vi "Lab Panel V5.26.vi"() -> ()   [LabVIEW 2017] (continued)
                n197 = call "sub vi - GET ALL TEMP v7.vi"("LA01-EN"=w245, "simulate"=w207, "LA02-EN"=w245, "LA03-EN"=w245, "LA04-EN"=w245, "LA05-EN"=w245, "Gen Cal Value"=1) -> ("ID"=w206:T24, "LA01 TEMP"=w243:T25, "LA02 TEMP"=w236:T25, "LA03 TEMP"=w229:T25, "LA04 TEMP"=w222:T25, "LA05 TEMP"=w215:T25)  [unwired: 1 in, 2 out]
                n198 = local write "LAB05 TEMP"(w215) -> ()
                n199 = local write "LAB04 TEMP"(w222) -> ()
                n200 = Unbundle(w229) -> ("T1"=w226:dbl, "T2"=w225:dbl, "T3"=w224:dbl, "T4"=w223:dbl)  [unwired: 2 out]
                n201 = Unbundle(w243) -> ("T1"=w241:dbl, "T2"=w240:dbl, "T3"=w239:dbl, "T4"=w238:dbl)  [unwired: 2 out]
                n202 = Unbundle(w236) -> ("T1"=w233:dbl, "T2"=w232:dbl, "T3"=w231:dbl, "T4"=w230:dbl)  [unwired: 2 out]
                n203 = Unbundle(w222) -> ("T1"=w220:dbl, "T2"=w219:dbl, "T3"=w218:dbl, "T4"=w217:dbl)  [unwired: 2 out]
                n204 = Unbundle(w215) -> ("T1"=w213:dbl, "T2"=w212:dbl, "T3"=w211:dbl, "T4"=w210:dbl)  [unwired: 2 out]
                n205 = local write "LAB01 TEMP"(w243) -> ()
                n206 = local write "LAB02 TEMP"(w236) -> ()
                n207 = local write "LAB03 TEMP"(w229) -> ()
                n208 = Unbundle(w206) -> ("id1"=→"LAB01-TP":bool, "id2"=→"LAB02-TP":bool, "id3"=→"LAB03-TP":bool, "id4"=→"LAB04-TP":bool, "id5"=→"LAB05-TP":bool)
                n209 = local read "TEMP LA05"() -> (w214:T9)
                n210 = local read "TEMP LA04"() -> (w221:T9)
                n211 = local read "TEMP LA02"() -> (w235:T9)
                n212 = local read "TEMP LA03"() -> (w228:T9)
                n213 = local read "TEMP LA01"() -> (w242:T9)
                n214 = Bundle(cluster=w228, "TL-1"=w226, "TN-1"=w225, "TL-2"=w224, "TN-2"=w223) -> (w227:T9)  [unwired: 4 in]
                n215 = Bundle(cluster=w242, "TL-1"=w241, "TN-1"=w240, "TL-2"=w239, "TN-2"=w238) -> (w237:T9)  [unwired: 4 in]
                n216 = Bundle(cluster=w235, "TL-1"=w233, "TN-1"=w232, "TL-2"=w231, "TN-2"=w230) -> (w234:T9)  [unwired: 4 in]
                n217 = Bundle(cluster=w221, "TL-1"=w220, "TN-1"=w219, "TL-2"=w218, "TN-2"=w217) -> (w216:T9)  [unwired: 4 in]
                n218 = Bundle(cluster=w214, "TL-1"=w213, "TN-1"=w212, "TL-2"=w211, "TN-2"=w210) -> (w209:T9)  [unwired: 4 in]
                n219 = local write "TEMP LA03"(w227) -> ()
                n220 = local write "TEMP LA01"(w237) -> ()
                n221 = local write "TEMP LA02"(w234) -> ()
                n222 = local write "TEMP LA05"(w209) -> ()
                n223 = local write "TEMP LA04"(w216) -> ()
              }
            }
            frame #2 {
              w256 = 0
              n224 = local read "LAB01 TEMP"() -> (w258:T12)
              n225 = local read "SIG LAB01-2"() -> (w253:T2)
              n226 = Unbundle By Name(w258) -> ("T1 Live"=w251:dbl, "T1 Neut"=w250:dbl, "T2 Live"=w249:dbl, "T2 Neut"=w248:dbl)  [unwired: 2 out]
              n227 = local read "SIG LAB01-1"() -> (w255:T2)
              n228 = local read "TEMP LA01"() -> (w259:T9)
              n229 = Bundle By Name(cluster=w259, "TL-1"=w251, "TN-1"=w250, "TL-2"=w249, "TN-2"=w248, "TL -1COUNT"=w256, "TN-1 COUNT"=w256, "TL-2 COUNT"=w256, "TN-2 COUNT"=w256) -> (w257:T9)
              n230 = Bundle(cluster=w255, "Tmp Live"=w251, "Tmp Neut"=w250) -> (w254:T2)  [unwired: 3 in]
              n231 = Bundle(cluster=w253, "Tmp Live"=w249, "Tmp Neut"=w248) -> (w252:T2)  [unwired: 3 in]
              n232 = local write "SIG LAB01-2"(w252) -> ()
              n233 = local write "SIG LAB01-1"(w254) -> ()
              n234 = local write "TEMP LA01"(w257) -> ()
            }
            frame #3 {
              w268 = 0
              n235 = local read "LAB02 TEMP"() -> (w270:T12)
              n236 = Unbundle By Name(w270) -> ("T1 Live"=w263:dbl, "T1 Neut"=w262:dbl, "T2 Live"=w261:dbl, "T2 Neut"=w260:dbl)  [unwired: 2 out]
              n237 = local read "SIG LAB02-1"() -> (w267:T2)
              n238 = local read "SIG LAB02-2"() -> (w266:T2)
              n239 = local read "TEMP LA02"() -> (w271:T9)
              n240 = Bundle By Name(cluster=w271, "TL-1"=w263, "TN-1"=w262, "TL-2"=w261, "TN-2"=w260, "TL -1COUNT"=w268, "TN-1 COUNT"=w268, "TL-2 COUNT"=w268, "TN-2 COUNT"=w268) -> (w269:T9)
              n241 = Bundle(cluster=w266, "Tmp Live"=w261, "Tmp Neut"=w260) -> (w264:T2)  [unwired: 3 in]
              n242 = Bundle(cluster=w267, "Tmp Live"=w263, "Tmp Neut"=w262) -> (w265:T2)  [unwired: 3 in]
              n243 = local write "TEMP LA02"(w269) -> ()
              n244 = local write "SIG LAB02-1"(w265) -> ()
              n245 = local write "SIG LAB02-2"(w264) -> ()
            }
            frame #4 {
              w280 = 0
              n246 = local read "LAB03 TEMP"() -> (w282:T12)
              n247 = Unbundle By Name(w282) -> ("T1 Live"=w275:dbl, "T1 Neut"=w274:dbl, "T2 Live"=w273:dbl, "T2 Neut"=w272:dbl)  [unwired: 2 out]
              n248 = local read "SIG LAB03-1"() -> (w279:T2)
              n249 = local read "SIG LAB03-2"() -> (w278:T2)
              n250 = local read "TEMP LA03"() -> (w283:T9)
              n251 = Bundle By Name(cluster=w283, "TL-1"=w275, "TN-1"=w274, "TL-2"=w273, "TN-2"=w272, "TL -1COUNT"=w280, "TN-1 COUNT"=w280, "TL-2 COUNT"=w280, "TN-2 COUNT"=w280) -> (w281:T9)
              n252 = Bundle(cluster=w278, "Tmp Live"=w273, "Tmp Neut"=w272) -> (w276:T2)  [unwired: 3 in]
              n253 = Bundle(cluster=w279, "Tmp Live"=w275, "Tmp Neut"=w274) -> (w277:T2)  [unwired: 3 in]
              n254 = local write "TEMP LA03"(w281) -> ()
              n255 = local write "SIG LAB03-2"(w276) -> ()
              n256 = local write "SIG LAB03-1"(w277) -> ()
            }
            frame #5 {
              w292 = 0
              n257 = local read "LAB04 TEMP"() -> (w294:T12)
              n258 = Unbundle By Name(w294) -> ("T1 Live"=w287:dbl, "T1 Neut"=w286:dbl, "T2 Live"=w285:dbl, "T2 Neut"=w284:dbl)  [unwired: 2 out]
              n259 = local read "SIG LAB04-2"() -> (w290:T2)
              n260 = local read "SIG LAB04-1"() -> (w291:T2)
              n261 = local read "TEMP LA04"() -> (w295:T9)
              n262 = Bundle By Name(cluster=w295, "TL-1"=w287, "TN-1"=w286, "TL-2"=w285, "TN-2"=w284, "TL -1COUNT"=w292, "TN-1 COUNT"=w292, "TL-2 COUNT"=w292, "TN-2 COUNT"=w292) -> (w293:T9)
              n263 = Bundle(cluster=w290, "Tmp Live"=w285, "Tmp Neut"=w284) -> (w288:T2)  [unwired: 3 in]
              n264 = Bundle(cluster=w291, "Tmp Live"=w287, "Tmp Neut"=w286) -> (w289:T2)  [unwired: 3 in]
              n265 = local write "SIG LAB04-2"(w288) -> ()
              n266 = local write "TEMP LA04"(w293) -> ()
              n267 = local write "SIG LAB04-1"(w289) -> ()
            }
            frame #6 {
              w304 = 0
              n268 = local read "LAB05 TEMP"() -> (w306:T12)
              n269 = Unbundle By Name(w306) -> ("T1 Live"=w299:dbl, "T1 Neut"=w298:dbl, "T2 Live"=w297:dbl, "T2 Neut"=w296:dbl)  [unwired: 2 out]
              n270 = local read "SIG LAB05-2"() -> (w302:T2)
              n271 = local read "SIG LAB05-1"() -> (w303:T2)
              n272 = local read "TEMP LA05"() -> (w307:T9)
              n273 = Bundle By Name(cluster=w307, "TL-1"=w299, "TN-1"=w298, "TL-2"=w297, "TN-2"=w296, "TL -1COUNT"=w304, "TN-1 COUNT"=w304, "TL-2 COUNT"=w304, "TN-2 COUNT"=w304) -> (w305:T9)
              n274 = Bundle(cluster=w302, "Tmp Live"=w297, "Tmp Neut"=w296) -> (w300:T2)  [unwired: 3 in]
              n275 = Bundle(cluster=w303, "Tmp Live"=w299, "Tmp Neut"=w298) -> (w301:T2)  [unwired: 3 in]
              n276 = local write "SIG LAB05-2"(w300) -> ()
              n277 = local write "SIG LAB05-1"(w301) -> ()
              n278 = local write "TEMP LA05"(w305) -> ()
            }
          }
        }
        frame #11 {
          # "create analog task"
          n279 = local read "Simulate"() -> (w308:bool)
          n280 = case shown="False" w308 {
            frame False {
              n281 = local read "SAMPLES"() -> (w310:dbl)
              n282 = local read "RATE (Hz)"() -> (w311:dbl)
              n283 = local read "AI Task0"() -> (w314:dbl)
              n284 = local read "AI Task2"() -> (w312:dbl)
              n285 = local read "AI Task1"() -> (w313:dbl)
              n286 = call "sub vi - AI USB4704 (3)  Create Task v4.vi"(0:w314, 5:w313, 7:w312, "Rate Hz"=w311, "Samples"=w310) -> ("TASK USB 0"=→"AI Task0":i32, "TASK USB 1"=→"AI Task1":i32, "TASK USB 2"=→"AI Task2":i32, "AI Task Er"=w309:bool)  [unwired: 6 in, 1 out]
              n287 = local write "Reset Error"(w309) -> ()
              "AI Task" <- TRUE
            }
            frame True {
            }
          }
        }
        frame #12 {
          # "enable front panel, all settings done"
          n288 = property on="Tab Control 2" class="TabCtl (strict)"("DisabledEnum"=T16."Enabled" ("Disabled")) -> ()  [unwired: 2 in, 2 out]
          n289 = property on="Tab Control 2" class="TabCtl (strict)"("Value"=0) -> ()  [unwired: 2 in, 2 out]
        }
        frame #13 {
          n290 = property on="Tab Control 2" class="TabCtl (strict)"("Value"=0) -> ()  [unwired: 2 in, 2 out]
        }
      }
    }
    frame #2 {
      w322 = 250.0
      # "frames that only action on certain cycles, 13, 14, 15, 16, 19, 21"
      n291 = node-c288(w322) -> (w324:T18)  [unwired: 3 in]
      n292 = timed-loop {
        timing: w324 -> [_]
        timing-out: [_] -> w323
        tunnel: w322 -> [w325]
        i -> [w351]
        stop <- w326 stop-if-true
        n293 = node-c288() -> ()  [unwired: 1 in, 1 out]
        n294 = local read "Resets Done"() -> (w330:dbl)
        n295 = local read "SELECT LAB05-2"() -> (w331:T3)
        n296 = local read "SELECT LAB05-1"() -> (w332:T3)
        n297 = local read "SELECT LAB04-2"() -> (w333:T3)
        n298 = local read "SELECT LAB03-1"() -> (w336:T3)
        n299 = local read "SELECT LAB02-2"() -> (w337:T3)
        n300 = local read "SELECT LAB01-1"() -> (w340:T3)
        n301 = local read "SELECT LAB03-2"() -> (w335:T3)
        n302 = local read "SELECT LAB01-2"() -> (w339:T3)
        n303 = local read "SELECT LAB04-1"() -> (w334:T3)
        n304 = Greater?(x=w330, y=50) -> (0:w327:bool)
        n305 = local read "SELECT LAB02-1"() -> (w338:T3)
        n306 = local read "run lab03-2"() -> (w345:bool)
        n307 = local read "run lab04-1"() -> (w344:bool)
        n308 = local read "run lab05-1"() -> (w342:bool)
        n309 = local read "run lab04-2"() -> (w343:bool)
        n310 = local read "run lab05-2"() -> (w341:bool)
        n311 = local read "run lab03-1"() -> (w346:bool)
        n312 = local read "run lab02-2"() -> (w347:bool)
        n313 = local read "run lab02-1"() -> (w348:bool)
        n314 = local read "run lab01-1"() -> (w350:bool)
        n315 = local read "run lab01-2"() -> (w349:bool)
        n316 = Or(x=w327, y="stop") -> (x .or. y?=w326:bool)
        n317 = global write "Global display 1.vi" "stop disp"(w326) -> ()
        n318 = stacked-sequence {
          seq-local: [_ _ w430 _ _ _ _ _ _ _ _ _ _ _ _ _ _ _ _ _ _ _ _ _ _] -> [_ _ _ _ _ _ w2531 _ _ _ _ _ _ _ _ _ _ _ _ _ _ _ _ _ _]
          seq-local: [_ _ w429 _ _ _ _ _ _ _ _ _ _ _ _ _ _ _ _ _ _ _ _ _ _] -> [_ _ _ _ _ _ w2530 _ _ _ _ _ _ _ _ _ _ _ _ _ _ _ _ _ _]
          seq-local: [_ _ w416 _ _ _ _ _ _ _ _ _ _ _ _ _ _ _ _ _ _ _ _ _ _] -> [_ _ _ _ _ _ w2529 _ _ _ _ _ _ _ _ _ _ _ _ _ _ _ _ _ _]
          seq-local: [_ _ w415 _ _ _ _ _ _ _ _ _ _ _ _ _ _ _ _ _ _ _ _ _ _] -> [_ _ _ _ _ _ w2528 _ _ _ _ _ _ _ _ _ _ _ _ _ _ _ _ _ _]
          seq-local: [_ _ w414 _ _ _ _ _ _ _ _ _ _ _ _ _ _ _ _ _ _ _ _ _ _] -> [_ _ _ _ _ _ w2527 _ _ _ _ _ _ _ _ _ _ _ _ _ _ _ _ _ _]
          seq-local: [_ _ w413 _ _ _ _ _ _ _ _ _ _ _ _ _ _ _ _ _ _ _ _ _ _] -> [_ _ _ _ _ _ w2526 _ _ _ _ _ _ _ _ _ _ _ _ _ _ _ _ _ _]
          seq-local: [_ _ w412 _ _ _ _ _ _ _ _ _ _ _ _ _ _ _ _ _ _ _ _ _ _] -> [_ _ _ _ _ _ w2525 _ _ _ _ _ _ _ _ _ _ _ _ _ _ _ _ _ _]
          seq-local: [_ _ w411 _ _ _ _ _ _ _ _ _ _ _ _ _ _ _ _ _ _ _ _ _ _] -> [_ _ _ _ _ _ w2524 _ _ _ _ _ _ _ _ _ _ _ _ _ _ _ _ _ _]
          seq-local: [_ _ w410 _ _ _ _ _ _ _ _ _ _ _ _ _ _ _ _ _ _ _ _ _ _] -> [_ _ _ _ _ _ w2523 _ _ _ _ _ _ _ _ _ _ _ _ _ _ _ _ _ _]
          seq-local: [_ _ w409 _ _ _ _ _ _ _ _ _ _ _ _ _ _ _ _ _ _ _ _ _ _] -> [_ _ _ _ _ _ w2522 _ _ _ _ _ _ _ _ _ _ _ _ _ _ _ _ _ _]
          seq-local: [_ _ _ _ _ _ _ _ _ _ _ _ w3667 _ _ _ _ _ _ _ _ _ _ _ _] -> [_ _ _ _ _ _ _ _ _ _ _ _ _ w3705 _ _ _ _ _ _ _ _ _ _ _]
          tunnel: w350 -> [_ _ _ w446 w694 w2121 w2551 w2866 w3353 _ _ _ _ _ w3989 _ w4946 _ _ w5234 w5537 w5718 _ _ _]
          tunnel: w349 -> [_ _ _ w445 w692 w2120 w2550 w2867 w3352 _ _ _ _ _ w3988 _ w4944 _ _ w5233 w5536 w5716 _ _ _]
          tunnel: w348 -> [_ _ _ w444 w690 w2119 w2549 w2865 w3351 _ _ _ _ _ w3987 _ w4942 _ _ w5232 w5535 w5715 _ _ _]
          tunnel: w347 -> [_ _ _ w443 w688 w2118 w2548 w2864 w3350 _ _ _ _ _ w3986 _ w4940 _ _ w5231 w5534 w5714 _ _ _]
          tunnel: w346 -> [_ _ _ w442 w686 w2117 w2547 w2863 w3349 _ _ _ _ _ w3985 _ w4938 _ _ w5230 w5533 w5713 _ _ _]
          tunnel: w345 -> [_ _ _ w441 w684 w2116 w2546 w2862 w3348 _ _ _ _ _ w3984 _ w4936 _ _ w5229 w5532 w5712 _ _ _]
          tunnel: w344 -> [_ _ _ w440 w682 w2115 w2545 w2861 w3347 _ _ _ _ _ w3983 _ w4934 _ _ w5228 w5531 w5711 _ _ _]
          tunnel: w343 -> [_ _ _ w439 w680 w2114 w2544 w2860 w3346 _ _ _ _ _ w3982 _ w4932 _ _ w5227 w5530 w5710 _ _ _]
          tunnel: w342 -> [_ _ _ w438 w678 w2113 w2543 w2859 w3345 _ _ _ _ _ w3981 _ w4930 _ _ w5226 w5529 w5709 _ _ _]
          tunnel: w341 -> [_ _ _ w437 w676 w2112 w2542 w2858 w3344 _ _ _ _ _ w3980 _ w4928 _ _ w5225 w5528 w5708 _ _ _]
          tunnel: w340 -> [_ _ _ _ w693 w2111 w2541 _ _ _ _ _ _ _ _ _ w4948 _ _ _ _ _ w6062 _ _]
          tunnel: w339 -> [_ _ _ _ w691 w2110 w2540 _ _ _ _ _ _ _ _ _ w4943 _ _ _ _ _ w6061 _ _]
          tunnel: w338 -> [_ _ _ _ w689 w2109 w2539 _ _ _ _ _ _ _ _ _ w4941 _ _ _ _ _ w6060 _ _]
          tunnel: w337 -> [_ _ _ _ w687 w2108 w2538 _ _ _ _ _ _ _ _ _ w4939 _ _ _ _ _ w6059 _ _]
          tunnel: w336 -> [_ _ _ _ w685 w2107 w2537 _ _ _ _ _ _ _ _ _ w4937 _ _ _ _ _ w6058 _ _]
          tunnel: w335 -> [_ _ _ _ w683 w2106 w2536 _ _ _ _ _ _ _ _ _ w4935 _ _ _ _ _ w6057 _ _]
          tunnel: w334 -> [_ _ _ _ w681 w2105 w2535 _ _ _ _ _ _ _ _ _ w4933 _ _ _ _ _ w6056 _ _]
          tunnel: w333 -> [_ _ _ _ w679 w2104 w2534 _ _ _ _ _ _ _ _ _ w4931 _ _ _ _ _ w6055 _ _]
          tunnel: w332 -> [_ _ _ _ w677 w2103 w2533 _ _ _ _ _ _ _ _ _ w4929 _ _ _ _ _ w6054 _ _]
          tunnel: w331 -> [_ _ _ _ w675 w2102 w2532 _ _ _ _ _ _ _ _ _ w4927 _ _ _ _ _ w6053 _ _]
          tunnel: w327 -> [_ _ _ _ _ _ _ _ _ _ _ _ _ _ _ _ _ _ _ _ _ _ _ _ w6115]
          tunnel: w326 -> [_ _ _ _ _ _ _ _ _ _ _ _ _ _ _ _ _ _ _ _ _ _ _ _ w6114]
          tunnel: w325 -> [_ w366 _ _ _ _ _ _ _ _ _ _ _ _ _ _ _ _ _ _ _ _ _ _ _]
          frame #0 {
            n319 = local read "AI Task"() -> (w354:bool)
            n320 = global write "Global 1.vi" "RATE(Hz)"("RATE (Hz)") -> ()
            n321 = case shown="True" w354 {
              frame False {
              }
              frame True {
                n322 = local read "AI Task2"() -> (w362:dbl)
                n323 = local read "AI Task1"() -> (w363:dbl)
                n324 = local read "AI Task0"() -> (w364:dbl)
                n325 = call "sub vi - AI USB4704 (3) v73.vi"("Task0"=w364, "Task1"=w363, "Task2"=w362, "SAMPLES"="SAMPLES 2") -> ("data 0"=→"AI data 0" →"AI Data 0":waveform(dbl)[], "data 1"=→"AI data 1" →"AI Data 1":waveform(dbl)[], "data 2"=→"AI data 2" →"AI Data 2":waveform(dbl)[], "loop time"=→"AI loop time":dbl, "error array"=→"AI Error":errorcluster[])  [unwired: 7 in]
              }
            }
          }
          frame #1 {
            w373 = FALSE
            # "set up cycle control"
            n326 = local read "jig cycle"() -> (w377:dbl)
            n327 = local read "Amps Fail level"() -> (w371:dbl)
            n328 = local read "Simulate"() -> (w368:bool)
            n329 = Divide(x=w366, y=1000.0) -> (x/y=w365:dbl)
            n330 = Divide(x="JIG ON TIME (S)", y=w365) -> (x/y=→"on loops":dbl)
            n331 = Divide(x="JIG OFF TIME (S)", y=w365) -> (x/y=→"off loops":dbl)
            n332 = Increment(x=w377) -> (x+1=w376:dbl)
            n333 = local write "Simulate IND"(w368) -> ()
            n334 = global write "Global display 3.vi" "Amps Fail"(w371) -> ()
            n335 = local write "TEMP"(w373) -> ()
            n336 = local write "AI"(w373) -> ()
            n337 = local read "Network Directory"() -> (w370:path)
            n338 = local write "jig cycle"(w376) -> ()
            n339 = call "sub vi - check network dir v2.vi"("PATH"=w370) -> ("error"=w369:bool)  [unwired: 10 in]
            n340 = local write "network error"(w369) -> ()
            n341 = global write "Global display 3.vi" "network drive"(w369) -> ()
            n342 = event shown="[1] \"ADMIN\": Value Change" {
              selector: _ -> [_ _]
              dyn-events: _ -> [_ _]
              timeout: 10 -> [_ _]
              event Timeout {
                n343 = event-data() -> ()  [unwired: 1 in, 3 out]
              }
              event "ADMIN": Value Change {
                n344 = event-data() -> ()  [unwired: 1 in, 6 out]
                n345 = stacked-sequence {
                  seq-local: [_ w381 _] -> [_ _ w382]
                  frame #0 {
                    n346 = global write "Global 1.vi" "password"("9949") -> ()
                  }
                  frame #1 {
                    n347 = call "sub vi - password 1.vi"() -> ("RESULT"=w381:bool)  [unwired: 11 in]
                  }
                  frame #2 {
                    w384 = FALSE
                    n348 = property on="Tab Control 2" class="TabCtl (strict)"() -> ("Pages"=w388:refnum<vi>[])  [unwired: 2 in, 2 out]
                    n349 = Select(t=TRUE, s=w382, f=w384) -> (s? t:f=w383:bool)
                    n350 = Index Array(array=w388, index=8) -> (element=w386:refnum<vi>)
                    n351 = property class="Page"(reference=w386, "PageVis"=w383) -> ()  [unwired: 1 in, 2 out]
                    n352 = local write "ADMIN"(w384) -> ()
                  }
                }
              }
            }
          }
          frame #2 {
            w426 = 60.0
            # "convert temperature rise minutes to cycles"
            n353 = local read "SET LAB05-2"() -> (w390:T5)
            n354 = local read "SET LAB05-1"() -> (w392:T5)
            n355 = local read "SET LAB04-2"() -> (w394:T5)
            n356 = local read "SET LAB01-1"() -> (w408:T5)
            n357 = local read "SET LAB01-2"() -> (w406:T5)
            n358 = local read "SET LAB02-2"() -> (w402:T5)
            n359 = local read "SET LAB04-1"() -> (w396:T5)
            n360 = local read "SET LAB03-1"() -> (w400:T5)
            n361 = local read "SET LAB03-2"() -> (w398:T5)
            n362 = local read "SET LAB02-1"() -> (w404:T5)
            n363 = local read "JIG OFF TIME (S)"() -> (w431:dbl)
            n364 = local read "JIG ON TIME (S)"() -> (w432:dbl)
            n365 = Unbundle(w390) -> ("T-RISE mins"=w389:dbl)  [unwired: 4 out]
            n366 = Unbundle(w392) -> ("T-RISE mins"=w391:dbl)  [unwired: 4 out]
            n367 = Unbundle(w408) -> ("T-RISE mins"=w407:dbl)  [unwired: 4 out]
            n368 = Unbundle(w394) -> ("T-RISE mins"=w393:dbl)  [unwired: 4 out]
            n369 = Unbundle(w406) -> ("T-RISE mins"=w405:dbl)  [unwired: 4 out]
            n370 = Unbundle(w404) -> ("T-RISE mins"=w403:dbl)  [unwired: 4 out]
            n371 = Unbundle(w396) -> ("T-RISE mins"=w395:dbl)  [unwired: 4 out]
            n372 = Unbundle(w402) -> ("T-RISE mins"=w401:dbl)  [unwired: 4 out]
            n373 = Unbundle(w398) -> ("T-RISE mins"=w397:dbl)  [unwired: 4 out]
            n374 = Unbundle(w400) -> ("T-RISE mins"=w399:dbl)  [unwired: 4 out]
            n375 = Add(x=w432, y=w431) -> (x+y=w425:dbl)
            n376 = Multiply(x=w426, y=w397) -> (x*y=w421:dbl)
            n377 = Multiply(x=w426, y=w395) -> (x*y=w420:dbl)
            n378 = Multiply(x=w426, y=w393) -> (x*y=w419:dbl)
            n379 = Multiply(x=w426, y=w391) -> (x*y=w418:dbl)
            n380 = Multiply(x=w426, y=w389) -> (x*y=w417:dbl)
            n381 = Multiply(x=w426, y=w405) -> (x*y=w427:dbl)
            n382 = Multiply(x=w426, y=w399) -> (x*y=w422:dbl)
            n383 = Multiply(x=w426, y=w407) -> (x*y=w428:dbl)
            n384 = Multiply(x=w426, y=w403) -> (x*y=w424:dbl)
            n385 = Multiply(x=w426, y=w401) -> (x*y=w423:dbl)
            n386 = Divide(x=w418, y=w425) -> (x/y=w410:dbl)
            n387 = Divide(x=w419, y=w425) -> (x/y=w411:dbl)
            n388 = Divide(x=w420, y=w425) -> (x/y=w412:dbl)
            n389 = Divide(x=w417, y=w425) -> (x/y=w409:dbl)
            n390 = Divide(x=w422, y=w425) -> (x/y=w414:dbl)
            n391 = Divide(x=w428, y=w425) -> (x/y=w430:dbl)
            n392 = Divide(x=w427, y=w425) -> (x/y=w429:dbl)
            n393 = Divide(x=w424, y=w425) -> (x/y=w416:dbl)
            n394 = Divide(x=w423, y=w425) -> (x/y=w415:dbl)
            n395 = Divide(x=w421, y=w425) -> (x/y=w413:dbl)
          }
          frame #3 {
            # "control cycle loops"
            n396 = local read "JIG OFF TIME (S)"() -> (w435:dbl)
            n397 = local read "JIG ON TIME (S)"() -> (w434:dbl)
            n398 = local read "jig cycle"() -> (w448:dbl)
            n399 = local read "on loops"() -> (w450:dbl)
            n400 = local read "off loops"() -> (w449:dbl)
            n401 = Add(x=w435, y=w434) -> (x+y=w433:dbl)
            n402 = Add(x=w450, y=w449) -> (x+y=w436:dbl)
            n403 = Greater Or Equal?(x=w448, y=w436) -> (x >= y?=w447:bool)
            n404 = case shown="True" w447 {
              tunnel: w446 -> [_ w484]
              tunnel: w445 -> [_ w483]
              tunnel: w444 -> [_ w482]
              tunnel: w443 -> [_ w481]
              tunnel: w442 -> [_ w480]
              tunnel: w441 -> [_ w479]
              tunnel: w440 -> [_ w478]
              tunnel: w439 -> [_ w477]
              tunnel: w438 -> [_ w476]
              tunnel: w437 -> [_ w475]
              tunnel: w433 -> [_ w474]
              frame False {
              }
              frame True {
                # "increment cycle value and convert cycles to minutes for temp rise"
                n405 = stacked-sequence {
                  frame #0 {
                    n406 = local read "Temp read loop"() -> (w487:dbl)
                    n407 = Increment(x=w487) -> (x+1=w486:dbl)
                    n408 = local write "Temp read loop"(w486) -> ()
                  }
                  frame #1 {
                    n409 = local read "Temp read loop"() -> (w488:dbl)
                    n410 = Greater?(x=w488, y=20) -> (0:w490:bool)
                    n411 = case shown="True" w490 {
                      frame False {
                      }
                      frame True {
                        n412 = local write "Temp read loop"(1) -> ()
                      }
                    }
                  }
                }
                n413 = local read "JIG RELAY CYCLES"() -> (w473:T8)
                n414 = local read "Temp read loop"() -> (→"Tp Up":dbl)
                n415 = Unbundle By Name(w473) -> ("LAB01-1"=w471:dbl, "LAB01-2"=w469:dbl, "LAB02-1"=w467:dbl, "LAB02-2"=w465:dbl, "LAB03-1"=w463:dbl, "LAB03-2"=w461:dbl, "LAB04-1"=w459:dbl, "LAB04-2"=w457:dbl, "LAB05-1"=w455:dbl, "LAB05-2"=w453:dbl)
                n416 = stacked-sequence {
                  tunnel: w484 -> [w502 _ _ _ _ _ _ _ _ _]
                  tunnel: w483 -> [_ w519 _ _ _ _ _ _ _ _]
                  tunnel: w482 -> [_ _ w536 _ _ _ _ _ _ _]
                  tunnel: w481 -> [_ _ _ w553 _ _ _ _ _ _]
                  tunnel: w480 -> [_ _ _ _ w570 _ _ _ _ _]
                  tunnel: w479 -> [_ _ _ _ _ w587 _ _ _ _]
                  tunnel: w478 -> [_ _ _ _ _ _ w604 _ _ _]
                  tunnel: w477 -> [_ _ _ _ _ _ _ w621 _ _]
                  tunnel: w476 -> [_ _ _ _ _ _ _ _ w638 _]
                  tunnel: w475 -> [_ _ _ _ _ _ _ _ _ w655]
                  tunnel: w474 -> [w499 w516 w533 w550 w567 w584 w601 w618 w635 w652]
                  tunnel: w471 -> [w493 _ _ _ _ _ _ _ _ _]
                  tunnel: [w492 _ _ _ _ _ _ _ _ _] -> w470
                  tunnel: w469 -> [_ w510 _ _ _ _ _ _ _ _]
                  tunnel: [_ w509 _ _ _ _ _ _ _ _] -> w468
                  tunnel: w467 -> [_ _ w527 _ _ _ _ _ _ _]
                  tunnel: [_ _ w526 _ _ _ _ _ _ _] -> w466
                  tunnel: w465 -> [_ _ _ w544 _ _ _ _ _ _]
                  tunnel: [_ _ _ w543 _ _ _ _ _ _] -> w464
                  tunnel: w463 -> [_ _ _ _ w561 _ _ _ _ _]
                  tunnel: [_ _ _ _ w560 _ _ _ _ _] -> w462
                  tunnel: w461 -> [_ _ _ _ _ w578 _ _ _ _]
                  tunnel: [_ _ _ _ _ w577 _ _ _ _] -> w460
                  tunnel: w459 -> [_ _ _ _ _ _ w595 _ _ _]
                  tunnel: [_ _ _ _ _ _ w594 _ _ _] -> w458
                  tunnel: w457 -> [_ _ _ _ _ _ _ w612 _ _]
                  tunnel: [_ _ _ _ _ _ _ w611 _ _] -> w456
                  tunnel: w455 -> [_ _ _ _ _ _ _ _ w629 _]
                  tunnel: [_ _ _ _ _ _ _ _ w628 _] -> w454
                  tunnel: w453 -> [_ _ _ _ _ _ _ _ _ w646]
                  tunnel: [_ _ _ _ _ _ _ _ _ w645] -> w452
                  frame #0 {
                    n417 = local read "DISP LAB01-1"() -> (w497:T4)
                    n418 = Unbundle(w497) -> ("CYCLE"=w498:dbl)  [unwired: 2 out]
                    n419 = case shown="True" w502 {
                      tunnel: w498 -> [w504 w508]
                      tunnel: [w504 w507] -> w496
                      tunnel: w493 -> [w503 w506]
                      tunnel: [w503 w505] -> w492
                      frame False {
                      }
                      frame True {
                        n420 = Increment(x=w506) -> (x+1=w505:dbl)
                        n421 = Increment(x=w508) -> (x+1=w507:dbl)
                      }
                    }
                    n422 = Multiply(x=w496, y=w499) -> (x*y=w500:dbl)
                    n423 = Divide(x=w500, y=60.0) -> (x/y=w495:dbl)
                    n424 = Bundle(cluster=w497, "CYCLE"=w496, "MINS"=w495) -> (w494:T4)  [unwired: 1 in]
                    n425 = local write "DISP LAB01-1"(w494) -> ()
                  }
                  frame #1 {
                    n426 = local read "DISP LAB01-2"() -> (w514:T4)
                    n427 = Unbundle(w514) -> ("CYCLE"=w515:dbl)  [unwired: 2 out]
                    n428 = case shown="True" w519 {
                      tunnel: w515 -> [w521 w525]
                      tunnel: [w521 w524] -> w512
                      tunnel: w510 -> [w520 w523]
                      tunnel: [w520 w522] -> w509
                      frame False {
                      }
                      frame True {
                        n429 = Increment(x=w523) -> (x+1=w522:dbl)
                        n430 = Increment(x=w525) -> (x+1=w524:dbl)
                      }
                    }
                    n431 = Multiply(x=w512, y=w516) -> (x*y=w517:dbl)
                    n432 = Divide(x=w517, y=60.0) -> (x/y=w511:dbl)
                    n433 = Bundle(cluster=w514, "CYCLE"=w512, "MINS"=w511) -> (w513:T4)  [unwired: 1 in]
                    n434 = local write "DISP LAB01-2"(w513) -> ()
                  }
                  frame #2 {
                    n435 = local read "DISP LAB02-1"() -> (w531:T4)
                    n436 = Unbundle(w531) -> ("CYCLE"=w532:dbl)  [unwired: 2 out]
                    n437 = case shown="True" w536 {
                      tunnel: [w538 w542] -> w529
                      tunnel: w532 -> [w538 w541]
                      tunnel: w527 -> [w537 w540]
                      tunnel: [w537 w539] -> w526
                      frame False {
                      }
                      frame True {
                        n438 = Increment(x=w540) -> (x+1=w539:dbl)
                        n439 = Increment(x=w541) -> (x+1=w542:dbl)
                      }
                    }
                    n440 = Multiply(x=w529, y=w533) -> (x*y=w534:dbl)
                    n441 = Divide(x=w534, y=60.0) -> (x/y=w528:dbl)
                    n442 = Bundle(cluster=w531, "CYCLE"=w529, "MINS"=w528) -> (w530:T4)  [unwired: 1 in]
                    n443 = local write "DISP LAB02-1"(w530) -> ()
                  }
                  frame #3 {
                    n444 = local read "DISP LAB02-2"() -> (w548:T4)
                    n445 = Unbundle(w548) -> ("CYCLE"=w549:dbl)  [unwired: 2 out]
                    n446 = case shown="True" w553 {
                      tunnel: [w555 w559] -> w547
                      tunnel: w549 -> [w555 w558]
                      tunnel: w544 -> [w554 w557]
                      tunnel: [w554 w556] -> w543
                      frame False {
                      }
                      frame True {
                        n447 = Increment(x=w557) -> (x+1=w556:dbl)
                        n448 = Increment(x=w558) -> (x+1=w559:dbl)
                      }
                    }
                    n449 = Multiply(x=w547, y=w550) -> (x*y=w551:dbl)
                    n450 = Divide(x=w551, y=60.0) -> (x/y=w546:dbl)
                    n451 = Bundle(cluster=w548, "CYCLE"=w547, "MINS"=w546) -> (w545:T4)  [unwired: 1 in]
                    n452 = local write "DISP LAB02-2"(w545) -> ()
                  }
                  frame #4 {
                    n453 = local read "DISP LAB03-1"() -> (w565:T4)
                    n454 = Unbundle(w565) -> ("CYCLE"=w566:dbl)  [unwired: 2 out]
                    n455 = case shown="True" w570 {
                      tunnel: [w572 w576] -> w562
                      tunnel: w566 -> [w572 w575]
                      tunnel: w561 -> [w571 w574]
                      tunnel: [w571 w573] -> w560
                      frame False {
                      }
                      frame True {
                        n456 = Increment(x=w574) -> (x+1=w573:dbl)
                        n457 = Increment(x=w575) -> (x+1=w576:dbl)
                      }
                    }
                    n458 = Multiply(x=w562, y=w567) -> (x*y=w568:dbl)
                    n459 = Divide(x=w568, y=60.0) -> (x/y=w563:dbl)
                    n460 = Bundle(cluster=w565, "CYCLE"=w562, "MINS"=w563) -> (w564:T4)  [unwired: 1 in]
                    n461 = local write "DISP LAB03-1"(w564) -> ()
                  }
                  frame #5 {
                    n462 = local read "DISP LAB03-2"() -> (w582:T4)
                    n463 = Unbundle(w582) -> ("CYCLE"=w583:dbl)  [unwired: 2 out]
                    n464 = case shown="True" w587 {
                      tunnel: [w589 w593] -> w581
                      tunnel: w583 -> [w589 w592]
                      tunnel: w578 -> [w588 w591]
                      tunnel: [w588 w590] -> w577
                      frame False {
                      }
                      frame True {
                        n465 = Increment(x=w591) -> (x+1=w590:dbl)
                        n466 = Increment(x=w592) -> (x+1=w593:dbl)
                      }
                    }
                    n467 = Multiply(x=w581, y=w584) -> (x*y=w585:dbl)
                    n468 = Divide(x=w585, y=60.0) -> (x/y=w580:dbl)
                    n469 = Bundle(cluster=w582, "CYCLE"=w581, "MINS"=w580) -> (w579:T4)  [unwired: 1 in]
                    n470 = local write "DISP LAB03-2"(w579) -> ()
                  }
                  frame #6 {
                    n471 = local read "DISP LAB04-1"() -> (w599:T4)
                    n472 = Unbundle(w599) -> ("CYCLE"=w600:dbl)  [unwired: 2 out]
                    n473 = case shown="True" w604 {
                      tunnel: [w606 w610] -> w597
                      tunnel: w600 -> [w606 w609]
                      tunnel: w595 -> [w605 w608]
                      tunnel: [w605 w607] -> w594
                      frame False {
                      }
                      frame True {
                        n474 = Increment(x=w608) -> (x+1=w607:dbl)
                        n475 = Increment(x=w609) -> (x+1=w610:dbl)
                      }
                    }
                    n476 = Multiply(x=w597, y=w601) -> (x*y=w602:dbl)
                    n477 = Divide(x=w602, y=60.0) -> (x/y=w596:dbl)
                    n478 = Bundle(cluster=w599, "CYCLE"=w597, "MINS"=w596) -> (w598:T4)  [unwired: 1 in]
                    n479 = local write "DISP LAB04-1"(w598) -> ()
                  }
                  frame #7 {
                    n480 = local read "DISP LAB04-2"() -> (w616:T4)
                    n481 = Unbundle(w616) -> ("CYCLE"=w617:dbl)  [unwired: 2 out]
                    n482 = case shown="True" w621 {
                      tunnel: [w623 w627] -> w614
                      tunnel: w617 -> [w623 w626]
                      tunnel: w612 -> [w622 w625]
                      tunnel: [w622 w624] -> w611
                      frame False {
                      }
                      frame True {
                        n483 = Increment(x=w625) -> (x+1=w624:dbl)
                        n484 = Increment(x=w626) -> (x+1=w627:dbl)
                      }
                    }
                    n485 = Multiply(x=w614, y=w618) -> (x*y=w620:dbl)
                    n486 = Divide(x=w620, y=60.0) -> (x/y=w613:dbl)
                    n487 = Bundle(cluster=w616, "CYCLE"=w614, "MINS"=w613) -> (w615:T4)  [unwired: 1 in]
                    n488 = local write "DISP LAB04-2"(w615) -> ()
                  }
                  frame #8 {
                    n489 = local read "DISP LAB05-1"() -> (w633:T4)
                    n490 = Unbundle(w633) -> ("CYCLE"=w634:dbl)  [unwired: 2 out]
                    n491 = case shown="True" w638 {
                      tunnel: [w640 w644] -> w631
                      tunnel: w634 -> [w640 w643]
                      tunnel: w629 -> [w639 w642]
                      tunnel: [w639 w641] -> w628
                      frame False {
                      }
                      frame True {
                        n492 = Increment(x=w642) -> (x+1=w641:dbl)
                        n493 = Increment(x=w643) -> (x+1=w644:dbl)
                      }
                    }
                    n494 = Multiply(x=w631, y=w635) -> (x*y=w636:dbl)
                    n495 = Divide(x=w636, y=60.0) -> (x/y=w630:dbl)
                    n496 = Bundle(cluster=w633, "CYCLE"=w631, "MINS"=w630) -> (w632:T4)  [unwired: 1 in]
                    n497 = local write "DISP LAB05-1"(w632) -> ()
                  }
                  frame #9 {
                    n498 = local read "DISP LAB05-2"() -> (w651:T4)
                    n499 = Unbundle(w651) -> ("CYCLE"=w650:dbl)  [unwired: 2 out]
                    n500 = case shown="True" w655 {
                      tunnel: [w657 w661] -> w649
                      tunnel: w650 -> [w657 w660]
                      tunnel: w646 -> [w656 w659]
                      tunnel: [w656 w658] -> w645
                      frame False {
                      }
                      frame True {
                        n501 = Increment(x=w659) -> (x+1=w658:dbl)
                        n502 = Increment(x=w660) -> (x+1=w661:dbl)
                      }
                    }
                    n503 = Multiply(x=w649, y=w652) -> (x*y=w653:dbl)
                    n504 = Divide(x=w653, y=60.0) -> (x/y=w648:dbl)
                    n505 = Bundle(cluster=w651, "CYCLE"=w649, "MINS"=w648) -> (w647:T4)  [unwired: 1 in]
                    n506 = local write "DISP LAB05-2"(w647) -> ()
                  }
                }
                n507 = local write "jig cycle"(0) -> ()
                n508 = Bundle By Name(cluster=w473, "LAB01-1"=w470, "LAB01-2"=w468, "LAB02-1"=w466, "LAB02-2"=w464, "LAB03-1"=w462, "LAB03-2"=w460, "LAB04-1"=w458, "LAB04-2"=w456, "LAB05-1"=w454, "LAB05-2"=w452) -> (w472:T8)
                n509 = local write "JIG RELAY CYCLES"(w472) -> ()
              }
            }
          }
          frame #4 {
            # "START & STOP test RUN switch change, start test if true and stop test if false"
            n510 = Get Date/Time In Seconds() -> (seconds since 1Jan1904=w673:timestamp)
            n511 = local read "C drive data root dir"() -> (w666:path)
            n512 = Format Date/Time String(time format string (%c)="%b\\%a%d", seconds (now)=w673) -> (date/time string=w697:string)  [unwired: 1 in]
            n513 = Format Date/Time String(time format string (%c)="%H%M", seconds (now)=w673) -> (date/time string=w695:string)  [unwired: 1 in]
            n514 = Format Date/Time String(time format string (%c)="LabPanel%Y", seconds (now)=w673) -> (date/time string=w672:string)  [unwired: 1 in]
            n515 = Path To String(path=w666) -> (string=w669:string)
            n516 = global write "Global 1.vi" "C drive root path"(w666) -> ()
            n517 = local read "Ref deg C"() -> (w662:dbl)
            n518 = Concatenate Strings(w669, "\\") -> (w667:string)
            n519 = event shown="[1] \"RUN LAB01-1\": Value Change" {
              selector: _ -> [_ _ _ _ _ _ _ _ _ _ _]
              dyn-events: _ -> [_ _ _ _ _ _ _ _ _ _ _]
              timeout: 10 -> [_ _ _ _ _ _ _ _ _ _ _]
              tunnel: w667 -> [_ w710 w850 w991 w1131 w1271 w1411 w1551 w1691 w1831 w1972]
              tunnel: w697 -> [_ w709 w849 w990 w1130 w1270 w1410 w1550 w1690 w1830 w1971]
              tunnel: w695 -> [_ w707 w848 w989 w1129 w1269 w1409 w1549 w1689 w1829 w1970]
              tunnel: w693 -> [_ w708 _ _ _ _ _ _ _ _ _]
              tunnel: w694 -> [_ _ _ _ _ _ _ _ _ _ _]
              tunnel: w692 -> [_ _ _ _ _ _ _ _ _ _ _]
              tunnel: w691 -> [_ _ w847 _ _ _ _ _ _ _ _]
              tunnel: w690 -> [_ _ _ _ _ _ _ _ _ _ _]
              tunnel: w689 -> [_ _ _ w988 _ _ _ _ _ _ _]
              tunnel: w688 -> [_ _ _ _ _ _ _ _ _ _ _]
              tunnel: w687 -> [_ _ _ _ w1128 _ _ _ _ _ _]
              tunnel: w686 -> [_ _ _ _ _ _ _ _ _ _ _]
              tunnel: w685 -> [_ _ _ _ _ w1268 _ _ _ _ _]
              tunnel: w684 -> [_ _ _ _ _ _ _ _ _ _ _]
              tunnel: w683 -> [_ _ _ _ _ _ w1408 _ _ _ _]
              tunnel: w682 -> [_ _ _ _ _ _ _ _ _ _ _]
              tunnel: w681 -> [_ _ _ _ _ _ _ w1548 _ _ _]
              tunnel: w680 -> [_ _ _ _ _ _ _ _ _ _ _]
              tunnel: w679 -> [_ _ _ _ _ _ _ _ w1688 _ _]
              tunnel: w678 -> [_ _ _ _ _ _ _ _ _ _ _]
              tunnel: w677 -> [_ _ _ _ _ _ _ _ _ w1828 _]
              tunnel: w676 -> [_ _ _ _ _ _ _ _ _ _ _]
              tunnel: w675 -> [_ _ _ _ _ _ _ _ _ _ w1969]
              tunnel: w672 -> [_ w706 w846 w987 w1127 w1267 w1407 w1547 w1687 w1827 w1968]
              tunnel: [_ w705 w845 w986 w1126 w1266 w1406 w1546 w1686 w1826 w1967] -> w670
              tunnel: "RESET CYCLES TO ZERO?" -> [_ w704 w843 w984 w1124 w1264 w1404 w1544 w1684 w1824 w1965]
              tunnel: "YES" -> [_ w703 w842 w983 w1123 w1263 w1403 w1543 w1683 w1823 w1964]
              tunnel: "NO" -> [_ w702 w841 w982 w1122 w1262 w1402 w1542 w1682 w1822 w1963]
              tunnel: w662 -> [_ w699 w840 w980 w1121 w1261 w1401 w1541 w1681 w1821 w1961]
              event Timeout {
                n520 = event-data() -> ()  [unwired: 1 in, 3 out]
              }
              event "RUN LAB01-1": Value Change {
                n521 = event-data() -> ("NewVal"=w700:bool)  [unwired: 1 in, 5 out]
                n522 = local read "SIG LAB01-1"() -> (w701:T2)
                n523 = local write "run lab01-1"(w700) -> ()
                n524 = case shown="True" w700 {
                  tunnel: w710 -> [_ w748]
                  tunnel: w709 -> [_ w747]
                  tunnel: w708 -> [w712 w746]
                  tunnel: w707 -> [_ w745]
                  tunnel: w706 -> [_ w744]
                  tunnel: [w711 w743] -> w705
                  tunnel: w704 -> [_ w742]
                  tunnel: w703 -> [_ w741]
                  tunnel: w702 -> [_ w740]
                  tunnel: w701 -> [_ w739]
                  tunnel: w699 -> [_ w738]
                  frame False {
                    # "stop test"
                    n525 = stacked-sequence {
                      tunnel: w712 -> [_ w724 _]
                      tunnel: [_ w716 _] -> w711
                      frame #0 {
                        n526 = local read "DISP LAB01-1"() -> (w715:T4)
                        n527 = Bundle(cluster=w715, "STATUS"="STOP") -> (w713:T4)  [unwired: 2 in]
                        n528 = local write "DISP LAB01-1"(w713) -> ()
                      }
                      frame #1 {
                        n529 = local read "DISP LAB01-1"() -> (w723:T4)
                        n530 = Unbundle(w723) -> ("CYCLE"=w721:dbl, "MINS"=w722:dbl)  [unwired: 1 out]
                        n531 = case shown="\"CYCLE TEST\"" w724 {
                          tunnel: w722 -> [_ _ w731]
                          tunnel: w721 -> [w729 w730 _]
                          tunnel: [w729 w730 w731] -> w720
                          frame "CHART TEST", Default {
                          }
                          frame "CYCLE TEST" {
                          }
                          frame "T-RISE TEST" {
                          }
                        }
                        n532 = local read "TDMS LAB01-1"() -> (w728:refnum<k34>)
                        n533 = Build Array("STOPPED") -> (w725:string[])
                        n534 = Build Array(w720) -> (w719:dbl[])
                        n535 = TDMS Write(0:w728, 5:"TEST RESULT", 7:w725, 9:w719) -> (4:w717:refnum<k34>, 15:w718:errorcluster)  [unwired: 2 in, 2 out]
                        n536 = TDMS Close(8:w718, 11:w717) -> (0:w716:errorcluster)  [unwired: 1 out]
                      }
                      frame #2 {
                        n537 = stacked-sequence {
                          tunnel: "LAB01-1" -> [w734 w736]
                          frame #0 {
                            n538 = call "sub vi - defrag tdms v1.vi"("panel id"=w734) -> ("error out"=w733:errorcluster)  [unwired: 10 in]
                            n539 = local write "data file error"(w733) -> ()
                          }
                          frame #1 {
                            n540 = call "Save data file (stop) v3.vi"("panel id"=w736) -> ("network file save error"=w735:errorcluster)  [unwired: 9 in, 1 out]
                            n541 = local write "RESULT LAB01-1"(FALSE) -> ()
                            n542 = local write "data file error"(w735) -> ()
                          }
                        }
                      }
                    }
                  }
                  frame True {
                    n543 = stacked-sequence {
                      seq-local: [w750 _] -> [_ w754]
                      tunnel: w748 -> [_ w764]
                      tunnel: w747 -> [_ w763]
                      tunnel: w746 -> [_ w762]
                      tunnel: w745 -> [_ w761]
                      tunnel: w744 -> [_ w760]
                      tunnel: [_ w759] -> w743
                      tunnel: w742 -> [_ w758]
                      tunnel: w741 -> [_ w757]
                      tunnel: w740 -> [_ w756]
                      tunnel: w739 -> [w752 w755]
                      tunnel: w738 -> [_ w753]
                      frame #0 {
                        n544 = Unbundle(w752) -> ("AMPS"=w751:dbl)  [unwired: 4 out]
                        n545 = call "Check For Amps on v1.vi"("ID"="LAB01-1", "amps"=w751) -> ("amps"=w750:bool)  [unwired: 9 in]
                      }
                      frame #1 {
                        n546 = case shown="True" w754 {
                          tunnel: w764 -> [_ w777]
                          tunnel: w763 -> [_ w776]
                          tunnel: w762 -> [_ w775]
                          tunnel: w761 -> [_ w774]
                          tunnel: w760 -> [_ w773]
                          tunnel: [errorcluster {"status"=FALSE, "code"=0, "source"=""} ("error out") w772] -> w759
                          tunnel: w758 -> [_ w771]
                          tunnel: w757 -> [_ w770]
                          tunnel: w756 -> [_ w769]
                          tunnel: w755 -> [_ w768]
                          tunnel: w753 -> [_ w767]
                          frame False {
                            w765 = FALSE
                            n547 = local write "RUN LAB01-1"(w765) -> ()
                            n548 = local write "run lab01-1"(w765) -> ()
                          }
                          frame True {
                            n549 = stacked-sequence {
                              seq-local: [w778 _ _ _ _] -> [_ w799 _ _ _]
                              tunnel: w777 -> [w783 _ _ _ _]
                              tunnel: w776 -> [w779 _ _ _ _]
                              tunnel: w775 -> [w793 _ _ _ _]
                              tunnel: w774 -> [w786 _ _ _ _]
                              tunnel: w773 -> [w781 _ _ _ _]
                              tunnel: [_ w800 _ _ _] -> w772
                              tunnel: w771 -> [_ _ _ w821 _]
                              tunnel: w770 -> [_ _ _ w831 _]
                              tunnel: w769 -> [_ _ _ w830 _]
                              tunnel: w768 -> [_ _ _ _ _]
                              tunnel: w767 -> [_ _ _ _ w837]
                              frame #0 {
                                w780 = "\\"
                                n550 = case shown="\"CHART TEST\", Default" w793 {
                                tunnel: ["L01-1-CHART TEST-" "L01-1-CYCLE TEST-" "L01-1-T-RISE TEST-"] -> w789
                                frame "CHART TEST", Default {
                                }
                                frame "CYCLE TEST" {
                                }
                                frame "T-RISE TEST" {
                                }
                                }
                                n551 = local read "SET LAB01-1"() -> (w788:T5)
                                n552 = Unbundle(w788) -> ("DESCRIPTION"=w787:string)  [unwired: 4 out]
                                n553 = Concatenate Strings(w783, "\\", w781, w780, w779, w780) -> (w790:string)
                                n554 = String To Path(string=w790) -> (path=w792:path)
                                n555 = Concatenate Strings(w790, w789, w787, "-", w786, ".tdms") -> (w778:string)
                                n556 = Create Folder(path (use dialog)=w792) -> (error out=w791:errorcluster)  [unwired: 2 in, 2 out]
                                n557 = call <vilib>:"Clear Errors.vi"("error in (no error)"=w791) -> ()  [unwired: 5 in, 2 out]
                                n558 = global write "Global 1.vi" "LAB01-1 FILE"(w778) -> ()
                              }
                              frame #1 {
                                (unwired) FALSE
                                n559 = String To Path(string=w799) -> (path=w797:path)
                                n560 = TDMS Open(6:FALSE, 10:T21."create or replace" ("operation (0:open)"), 11:w797) -> (0:w800:errorcluster, 3:→"TDMS LAB01-1":refnum<k34>)  [unwired: 4 in]
                              }
                              frame #2 {
                                n561 = local read "TDMS LAB01-1"() -> (w819:refnum<k34>)
                                n562 = local read "SET LAB01-1"() -> (w808:T5)
                                n563 = Build Array("Testers Name", "Description", "Set Test Cycles", "T-Rise minutes", "T-Rise Deg C") -> (w809:string[])
                                n564 = Unbundle(w808) -> ("NAME"=w807:string, "DESCRIPTION"=w806:string, "CYCLES"=w805:dbl, "T-RISE mins"=w804:dbl, "T-RISE deg C"=w803:dbl)
                                n565 = Number To Decimal String(number=w805) -> (decimal integer string=w818:string)  [unwired: 1 in]
                                n566 = Number To Decimal String(number=w804) -> (decimal integer string=w817:string)  [unwired: 1 in]
                                n567 = Number To Decimal String(number=w803) -> (decimal integer string=w816:string)  [unwired: 1 in]
                                n568 = Build Array(w807, w806, w818, w817, w816) -> (w815:string[])
                                n569 = TDMS Set Properties(5:w815, 7:w809, 11:w819) -> ()  [unwired: 3 in, 4 out]
                              }
                              frame #3 {
                                n570 = local read "DISP LAB01-1"() -> (w829:T4)
                                n571 = Concatenate Strings("LAB01-1  ", w821) -> (w820:string)
                                n572 = Two Button Dialog(message=w820, 1:w830, 2:w831) -> (T button?=w823:bool)
                                n573 = case shown="True" w823 {
                                tunnel: w829 -> [w834 w835]
                                tunnel: [w834 w835] -> w828
                                tunnel: [w833 w836] -> w827
                                tunnel: [w832 w836] -> w826
                                frame False {
                                n574 = Unbundle(w834) -> ("CYCLE"=w833:dbl, "MINS"=w832:dbl)  [unwired: 1 out]
                                }
                                frame True {
                                w836 = 0.0
                                }
                                }
                                n575 = Bundle(cluster=w828, "CYCLE"=w827, "MINS"=w826, "STATUS"="RUN") -> (w825:T4)
                                n576 = local write "DISP LAB01-1"(w825) -> ()
                              }
                              frame #4 {
                                n577 = local read "TEMP START LAB01-1"() -> (w839:cluster{"TL":dbl, "TN":dbl})
                                n578 = Bundle(cluster=w839, "TL"=w837, "TN"=w837) -> (w838:cluster{"TL":dbl, "TN":dbl})
                                n579 = local write "TEMP START LAB01-1"(w838) -> ()
                              }
                            }
                          }
                        }
                      }
                    }
                  }
                }
              }
              event "RUN LAB01-2": Value Change {
                n580 = event-data() -> ("NewVal"=w844:bool)  [unwired: 1 in, 5 out]
                n581 = local write "run lab01-2"(w844) -> ()
                n582 = case shown="True" w844 {
                  tunnel: w850 -> [_ w888]
                  tunnel: w849 -> [_ w887]
                  tunnel: w847 -> [w852 w886]
                  tunnel: w848 -> [_ w885]
                  tunnel: w846 -> [_ w884]
                  tunnel: [w851 w883] -> w845
                  tunnel: w843 -> [_ w882]
                  tunnel: w842 -> [_ w881]
                  tunnel: w841 -> [_ w880]
                  tunnel: w840 -> [_ w878]
                  frame False {
                    # "stop test"
                    n583 = stacked-sequence {
                      tunnel: w852 -> [w861 _]
                      tunnel: [w853 _] -> w851
                      frame #0 {
                        n584 = local read "DISP LAB01-2"() -> (w860:T4)
                        n585 = Unbundle(w860) -> ("CYCLE"=w858:dbl, "MINS"=w859:dbl)  [unwired: 1 out]
                        n586 = case shown="\"CHART TEST\", Default" w861 {
